vi "RTPodPowerOn (1).vi"(8 "error in (no error)":errorcluster) -> (0 "error out":errorcluster, 1 "VISA Refnum out":refnum<visa-resource-name>)   [LabVIEW 2017]
doc: "Waits for the pod to be powered via a control on the Host front panel. If the manual shutoff is activated before, will give an error and proceed to RTShutdown.vi."
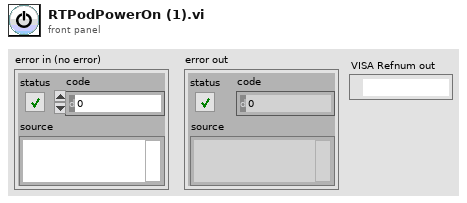
[diagram p1: front panel]
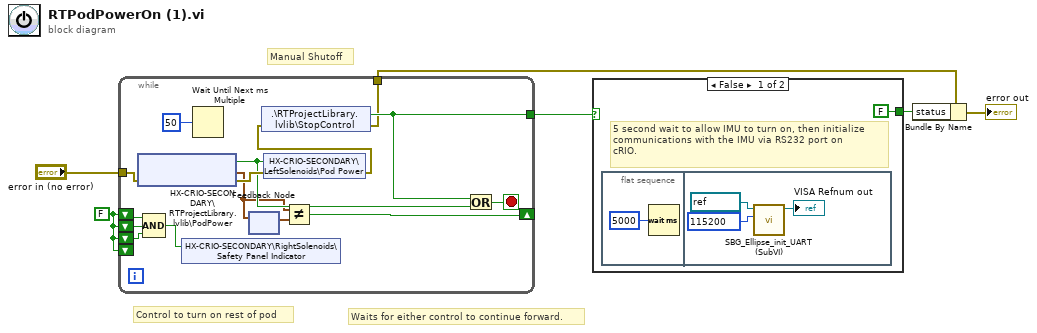
[diagram p0: block diagram]
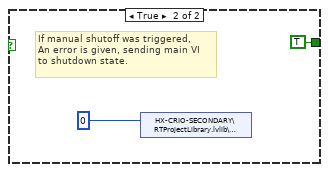
[diagram p2: hidden frame]
diagram:
  w1 = FALSE
  # "Waits for either control to continue forward."
  # "Control to turn on rest of pod"
  # "Manual Shutoff"
  n1 = while {
    tunnel: [w20] -> w3
    tunnel: "error in (no error)" -> [w16]
    tunnel: [w15] -> w4
    shift-right: [w11] -> _
    shift-left: w1 -> [w10]
    shift-left: w1 -> [w9]
    shift-left: w1 -> [w8]
    shift-left: w1 -> [_]
    stop <- w21 stop-if-true
    n2 = shared-variable "HX-CRIO-SECONDARY\\RTProjectLibrary.lvlib\\PodPower"(error in=w16) -> (w14:bool, error out=w18:errorcluster, w12:timestamp)
    n3 = Compound Arithmetic op=AND(w10, w9, w8) -> (w7:bool)
    n4 = shared-variable "HX-CRIO-SECONDARY\\RightSolenoids\\Safety Panel Indicator"(w7) -> ()  [unwired: 1 in, 1 out]
    n5 = Wait Until Next ms Multiple(millisecond multiple=u32 50 ("milliseconds to wait")) -> ()  [unwired: 1 out]
    n6 = feedback-in #1(w12) -> ()
    n7 = feedback #1() -> (w13:timestamp)  [unwired: 1 in]
    n8 = shared-variable "HX-CRIO-SECONDARY\\LeftSolenoids\\Pod Power"(w14, error in=w18) -> (error out=w17:errorcluster)
    n9 = shared-variable ".\\RTProjectLibrary.lvlib\\StopControl"(error in=w17) -> (w20:bool, error out=w15:errorcluster)
    n10 = Not Equal?(x=w12, y=w13) -> (x != y?=w11:bool)
    n11 = Or(x=w20, y=w14) -> (x .or. y?=w21:bool)
  }
  n12 = case shown="False" w3 {
    tunnel: [FALSE TRUE] -> w2
    frame False {
      # "5 second wait to allow IMU to turn on, then initialize\ncommunications with the IMU via RS232 port on\ncRIO."
      n13 = flat-sequence {
        frame #0 {
          n14 = Wait (ms)(milliseconds to wait=u32 5000) -> ()  [unwired: 1 out]
        }
        frame #1 {
          w25 = u32 115200 items=["9600"=9600, "19200"=19200, "36400"=36400, "57600"=57600, "115200"=115200, "230400"=230400, "460800"=460800, "921600"=921600] ("Baudrate")
          n15 = call "SBG_Ellipse_init_UART (SubVI).vi"("Baudrate"=w25, "VISA Refnum in"=refnum<visa-resource-name> "IMU" ("VISA resource name")) -> ("VISA Refnum out"=→"VISA Refnum out":refnum<visa-resource-name>)  [unwired: 8 in, 1 out]
        }
      }
    }
    frame True {
      # "If manual shutoff was triggered,\nAn error is given, sending main VI\nto shutdown state."
      n16 = shared-variable "HX-CRIO-SECONDARY\\RTProjectLibrary.lvlib\\CurrentState"(u8 0 ("CurrentState")) -> ()  [unwired: 1 in, 1 out]
    }
  }
  n17 = Bundle By Name(cluster=w4, "status"=w2) -> (→"error out":errorcluster)
